vi "Intensity Value.vi"(7 "intensity":i32=75, 8 "error in (no error)":errorcluster, 11 "VISA resource name":refnum<visa-resource-name>) -> (0 "error out":errorcluster, 2 "Connected? 2":bool, 3 "VISA resource name out":refnum<visa-resource-name>)   [LabVIEW 2018]
uses:
  <vilib>/Instr/_visa.llb/VISA Configure Serial Port (Instr).vi
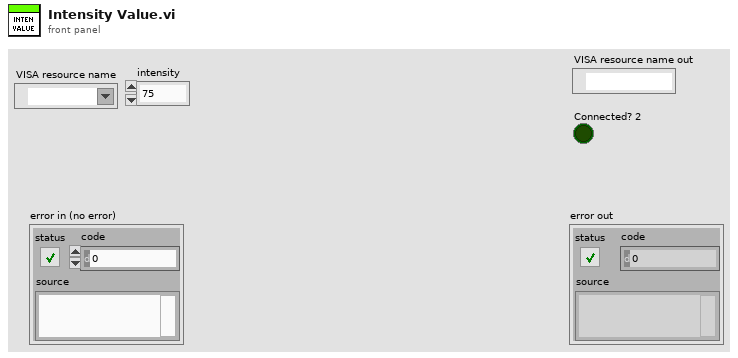
[diagram p1: front panel]
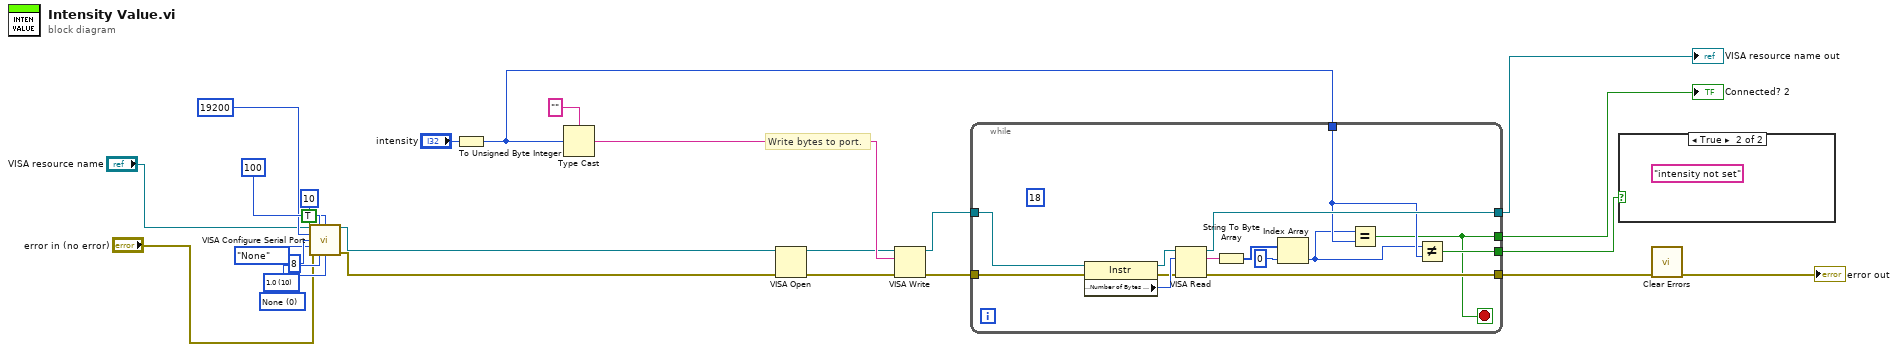
[diagram p0: block diagram]
diagram:
  w6 = u16 0 items=["None", "XON/XOFF", "RTS/CTS", "XON/XOFF & RTS/CTS", "DTR/DSR", "XON/XOFF & DTR/DSR"] ("flow control (0:none)")
  w7 = u16 10 items=["1.0"=10, "1.5"=15, "2.0"=20] ("stop bits (10: 1 bit)")
  # "Write bytes to port."
  n1 = call-poly "VISA Configure Serial Port"("VISA resource name"="VISA resource name", "timeout (10sec)"=u32 100, "termination char\n(0xA = '\\n' = LF)"=u8 10 ("termination char\n(0xA = '\\n' = LF)"), "Enable Termination\nChar (T)"=TRUE ("Enable Termination\nChar (T)"), "baud rate (9600)"=u32 19200, "data bits (8)"=u16 8, "parity (0:none)"=enum16{"None", "Odd", "Even", "Mark", "Space"}."None", "error in (no error)"="error in (no error)", "stop bits (10: 1 bit)"=w7, "flow control (0:none)"=w6) -> ("VISA resource name out"=w5:refnum<visa-resource-name>, "error out"=w3:errorcluster)  [unwired: 4 in]
  n2 = To Unsigned Byte Integer(number="intensity") -> (unsigned 8bit integer=w1:u8)
  n3 = Type Cast(type="", x=w1) -> (*(type *) &x=w21:string)
  n4 = VISA Open(error in (no error)=w3, VISA resource name=w5) -> (VISA resource name=w20:refnum<visa-resource-name>, error out=w19:errorcluster)  [unwired: 3 in]
  n5 = VISA Write(VISA resource name=w20, write buffer=w21, error in (no error)=w19) -> (VISA resource name out=w22:refnum<visa-resource-name>, error out=w23:errorcluster)  [unwired: 1 out]
  n6 = while {
    tunnel: [w39] -> w25
    tunnel: [w26] -> w24
    tunnel: w1 -> [w34]
    tunnel: w23 -> [w38]
    tunnel: [w36] -> w17
    tunnel: w22 -> [w37]
    tunnel: [w35] -> w16
    stop <- w26 stop-if-true
    (unwired) 18
    n7 = property class="Instr"(reference=w37, error in=w38) -> (reference out=w30:refnum<visa-resource-name>, error out=w28:errorcluster, "Serial Settings:Number of Bytes at Serial Port"=w29:u32)
    n8 = VISA Read(VISA resource name=w30, byte count=w29, error in (no error)=w28) -> (VISA resource name out=w35:refnum<visa-resource-name>, read buffer=w33:string, error out=w36:errorcluster)  [unwired: 1 out]
    n9 = String To Byte Array(string=w33) -> (unsigned byte array=w32:u8[])
    n10 = Index Array(array=w32, index=0) -> (element=w27:u8)
    n11 = Equal?(x=w27, y=w34) -> (x = y?=w26:bool)
    n12 = Not Equal?(x=w27, y=w34) -> (x != y?=w39:bool)
  }
  "Connected? 2" <- w24
  "VISA resource name out" <- w16
  n13 = case shown="True" w25 {
    frame False {
    }
    frame True {
      (unwired) "intensity not set"
    }
  }
  n14 = call <vilib>:"Clear Errors.vi"("error in (no error)"=w17) -> ("error out"=→"error out":errorcluster)  [unwired: 5 in, 1 out]
